vi "hdt_int_generator.vi"(9 "hdt.int.p.readParams":T2={"hdt.int.s.transferSource"=0, "hdt.int.p.useInternalMemStartPos"=FALSE, "hdt.int.p.memStartPos"=0.0, "hdt.int.p.readLength"=100, "hdt.int.p.readFwd"=TRUE, "hdt.int.p.memReadDec"=10, "hdt.int.p.startTransfer"=TRUE} {"hdt.int.s.transferSource" items=["memoryChan1", "memoryChan2", "processVarFixedNoPts", "processVarStream", "systemId", "interleaveMemCh1Ch2"]; "hdt.int.p.memReadDec" min=2}, 11 "hdt.int.p.memWriteSource":u8(ring) items=["ORT", "SICM"]) -> (0 "hdt.int.s.debug":T1)   [LabVIEW 2016]
uses:
  <vilib>/rvi/Emulation/niFpgaEmulationIsFPGAContextNoSignature.vi
  <vilib>/rvi/Emulation/niFpgaSctlEmulationGetInTimedLoop.vi
  <vilib>/rvi/errors/niFpgaSetErrorForExecOnDevCompSimple.vi
  <vilib>/rvi/eio/common/nirviEmuReportErrorAndStop.vi
  <vilib>/rvi/DataTransferAndStorage/Container/Common/niFpgaContainerGetUniqueNameForEmu.vi
  <vilib>/rvi/FIFO/Fifo_Resource/nirvififoEmulationSetSize.vi
  <vilib>/rvi/FIFO/Fifo_Resource/nirviFifoEmulationQueueMgr.vi
  <instcachedir>/0/nirviFifoEmulationQueueMgr_E5CAEC123FF24DC58D834DCA3CDAA9B5.lvgen/nirviFifoEmulationQueueMgr_E5CAEC123FF24DC58D834DCA3CDAA9B5_033.vi
  <vilib>/Utility/error.llb/Clear Errors.vi
  <vilib>/rvi/FIFO/Fifo_Resource/nirvififoEmulationCreateLock.vi
  <vilib>/rvi/Emulation/niFpgaProcessEmulError.vi
  <vilib>/rvi/FIFO/Fifo_Resource/nirvififoEmulationObtainLock.vi
  <vilib>/rvi/FIFO/Fifo_Resource/nirvififoEmulationReleaseLock.vi
  <vilib>/rvi/occurrence/nirviWaitOnOccurrenceBase.vi
  <vilib>/rvi/errors/nirviReportUnexpectedCaseInternalError.vi
  <vilib>/rvi/errors/nirviReportUnexpectedCaseInternalError (U32).vi
  <instcachedir>/0/nirviFifoEmulationQueueMgr_E5CAEC123FF24DC58D834DCA3CDAA9B5.lvgen/nirviFifoEmulationQueueMgr_E5CAEC123FF24DC58D834DCA3CDAA9B5_003.vi
  <vilib>/rvi/Memory/Memory_Emulation/nirvimemoryFastEmulation.vi
  <vilib>/rvi/Memory/Memory_Emulation/nirvimemoryEmulation.vi
  <instcachedir>/0/nirviFifoEmulationQueueMgr_E5CAEC123FF24DC58D834DCA3CDAA9B5.lvgen/nirviFifoEmulationQueueMgr_E5CAEC123FF24DC58D834DCA3CDAA9B5_009.vi
  <vilib>/rvi/FIFO/Fifo_Resource/nirvififoEmulationDetermineInputValidOut.vi
  <vilib>/rvi/DataTransferAndStorage/Container/XNode/niFpgaContainer.xnode
  <vilib>/rvi/FIFO/Fifo_Resource/nirvififoEmulationRead.vi
  <vilib>/rvi/DataTransferAndStorage/Handshake/Emulation/niFpgaHandshakeEmulation.vi
  <vilib>/rvi/FIFO/Fifo_Resource/nirvififoEmulationWrite.vi
  <instrlib>/_niInstr/Basic Elements/v1/FPGA/niInstr Basic Elements v1 FPGA.lvlib
panel:
  out "hdt.int.s.currentStagingEl":cluster{"Element":i16, "Output Valid":bool}
  out "hdt.int.s.storedMemPos":u16
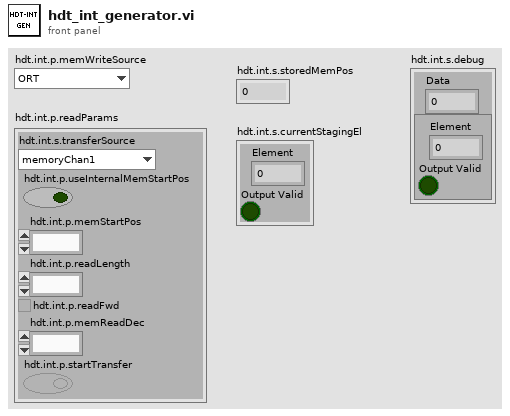
[diagram p1: front panel]
types:
  T1 = cluster{"Data":u16, cluster{"Element":i16, "Output Valid":bool}}
  T2 = cluster{"hdt.int.s.transferSource":u8, "hdt.int.p.useInternalMemStartPos":bool, "hdt.int.p.memStartPos":fxp<+,14,14>, "hdt.int.p.readLength":u16, "hdt.int.p.readFwd":bool, "hdt.int.p.memReadDec":u16, "hdt.int.p.startTransfer":bool}
  T3 = cluster{"Element":cluster{"address":u16, "interactionPair":cluster{"interaction":i16, "background":i16}}, "Output Valid":bool}
  T4 = cluster{"address":u16, "interactionPair":cluster{"interaction":i16, "background":i16}}
  T5 = cluster{"Element":cluster{"address":u16, "interactionPair":cluster{"interaction":i16, "background":i16}}, "Output Valid":bool}[]
  T6 = cluster{"interaction":i16, "Output Valid":bool}[]
  T7 = cluster{"Data":u16, cluster{"interaction":i16, "Output Valid":bool}}
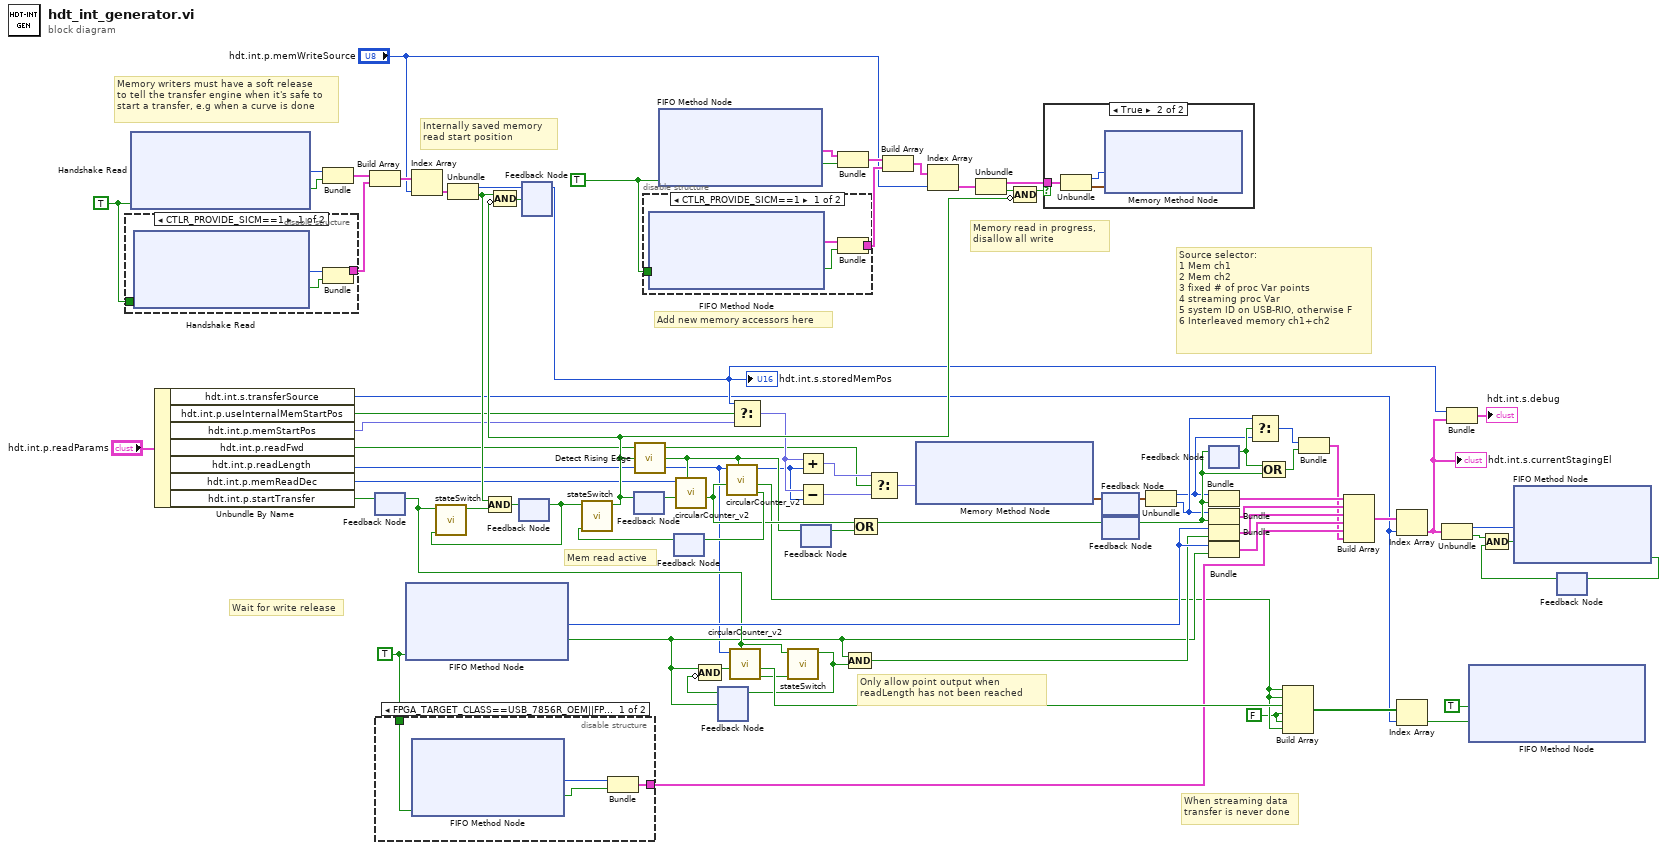
[diagram p0: block diagram]
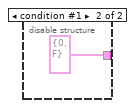
[diagram p2: hidden frame]
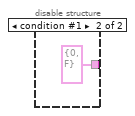
[diagram p3: hidden frame]
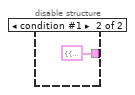
[diagram p4: hidden frame]
diagram:
  w3 = FALSE ("element")
  w45 = TRUE ("Ready for Output")
  w13 = TRUE ("Ready for Output")
  w46 = TRUE ("Ready for Output")
  # "Source selector:\n1 Mem ch1\n2 Mem ch2\n3 fixed # of proc Var points\n4 streaming proc Var\n5 system ID on USB-RIO, otherwise F\n6 Interleaved memory ch1+ch2"
  # "When streaming data\ntransfer is never done"
  # "Mem read active"
  # "Internally saved memory \nread start position"
  # "Memory writers must have a soft release\nto tell the transfer engine when it's safe to\nstart a transfer, e.g when a curve is done"
  # "Wait for write release"
  # "Only allow point output when readLength has not been reached"
  # "Memory read in progress,\ndisallow all write"
  # "Add new memory accessors here"
  n1 = disable-structure shown="CTLR_PROVIDE_SICM==1" {
    disable-tunnel: [w85 cluster{"Data":u16, "Output Valid":bool} {"Data"=0, "Output Valid"=FALSE}] -> w52
    disable-tunnel: w45 -> [w84 _]
    frame condition #0 (active) {
      n2 = xnode ("Handshake Read")("Ready for Output"=w84) -> ("Data"=w87:u16, "Output Valid"=w86:bool)  [unwired: 1 in, 1 out]
      n3 = Bundle("Data"=w87, "Output Valid"=w86) -> (w85:cluster{"Data":u16, "Output Valid":bool})  [unwired: 1 in]
    }
    frame condition #1 {
    }
  }
  n4 = xnode ("Handshake Read")("Ready for Output"=w45) -> ("Data"=w55:u16, "Output Valid"=w54:bool)  [unwired: 1 in, 1 out]
  n5 = Unbundle By Name("hdt.int.p.readParams") -> ("hdt.int.s.transferSource"=w30:u8, "hdt.int.p.useInternalMemStartPos"=w38:bool, "hdt.int.p.memStartPos"=w39:fxp<+,14,14>, "hdt.int.p.readFwd"=w15:bool, "hdt.int.p.readLength"=w14:u16, "hdt.int.p.memReadDec"=w37:u16, "hdt.int.p.startTransfer"=w36:bool)
  n6 = Bundle("Data"=w55, "Output Valid"=w54) -> (w53:cluster{"Data":u16, "Output Valid":bool})  [unwired: 1 in]
  n7 = Build Array(w53, w52) -> (w51:cluster{"Data":u16, "Output Valid":bool}[])
  n8 = feedback #1() -> (w24:bool)  [unwired: 1 in]
  n9 = feedback-in #1(w36) -> ()
  n10 = disable-structure shown="FPGA_TARGET_CLASS==USB_7856R_OEM||FPGA_TARGET_CLASS==USB_7856R" {
    disable-tunnel: w13 -> [w92 _]
    disable-tunnel: [w89 cluster{"Element":i16, "Output Valid":bool} {"Element"=0, "Output Valid"=FALSE} ("output cluster")] -> w12
    frame condition #0 (active) {
      n11 = xnode ("FIFO Method Node")("Ready for Output"=w92) -> ("Element"=w91:i16, "Output Valid"=w90:bool)  [unwired: 1 in, 1 out]
      n12 = Bundle("Element"=w91, "Output Valid"=w90) -> (w89:cluster{"Element":i16, "Output Valid":bool})  [unwired: 1 in]
    }
    frame condition #1 {
    }
  }
  n13 = xnode ("FIFO Method Node")("Ready for Output"=w13) -> ("Element"=w60:i16, "Output Valid"=w21:bool)  [unwired: 1 in, 1 out]
  n14 = Index Array(array=w51, index="hdt.int.p.memWriteSource") -> (element=w49:cluster{"Data":u16, "Output Valid":bool})
  n15 = Unbundle(w49) -> ("Data"=w48:u16, "Output Valid"=w43:bool)
  n16 = feedback #2() -> (w1:bool)  [unwired: 1 in]
  n17 = call "stateSwitch.vi"("disable"=w1, "enable"=w24) -> ("state"=w47:bool)  [unwired: 9 in]
  n18 = Compound Arithmetic op=AND(w43, w47) -> (w2:bool)
  n19 = feedback-in #2(w2) -> ()
  n20 = feedback #3() -> (w34:u16)  [unwired: 1 in]
  "hdt.int.s.storedMemPos" <- w34
  n21 = feedback #4() -> (w44:bool)  [unwired: 1 in]
  n22 = disable-structure shown="CTLR_PROVIDE_SICM==1" {
    disable-tunnel: [w95 T3 {"Element"={"address"=0, "interactionPair"={"interaction"=0, "background"=0}}, "Output Valid"=FALSE}] -> w75
    disable-tunnel: w46 -> [w94 _]
    frame condition #0 (active) {
      n23 = xnode ("FIFO Method Node")("Ready for Output"=w94) -> ("Element"=w97:T4, "Output Valid"=w96:bool)  [unwired: 1 in, 1 out]
      n24 = Bundle("Element"=w97, "Output Valid"=w96) -> (w95:T3)  [unwired: 1 in]
    }
    frame condition #1 {
    }
  }
  n25 = xnode ("FIFO Method Node")("Ready for Output"=w46) -> ("Element"=w82:T4, "Output Valid"=w81:bool)  [unwired: 1 in, 1 out]
  n26 = feedback #5() -> (w66:bool)  [unwired: 1 in]
  n27 = call "stateSwitch.vi"("disable"=w66, "enable"=w1) -> ("state"=w42:bool)  [unwired: 9 in]
  n28 = Compound Arithmetic op=AND(w43, invert w42) -> (w41:bool)
  n29 = feedback-in #3(w48, w41) -> ()
  n30 = feedback-in #4(w42) -> ()
  n31 = call <instrlib>:"Detect Rising Edge.vi"("signal"=w42) -> ("edge detected"=w26:bool)  [unwired: 14 in]
  n32 = call "circularCounter_v2.vi"("reset"=w26, "doStep"=w44, "maxCount"=w37) -> ("maxPulse"=w32:bool)  [unwired: 5 in, 3 out]
  n33 = feedback #6() -> (w57:bool)  [unwired: 1 in]
  n34 = Compound Arithmetic op=AND(w21, invert w57) -> (w58:bool)
  n35 = call "circularCounter_v2.vi"("reset"=w26, "doStep"=w32, "maxCount"=w14) -> ("maxReached"=w67:bool, "maxPulse"=w4:bool, "index"=w18:u16)  [unwired: 5 in, 1 out]
  n36 = feedback-in #5(w67) -> ()
  n37 = call "circularCounter_v2.vi"("reset"=w24, "doStep"=w58, "maxCount"=w14) -> ("maxReached"=w22:bool, "maxPulse"=w23:bool)  [unwired: 5 in, 2 out]
  n38 = Select(t=w34, s=w38, f=w39) -> (s? t:f=w19:fxp<+,16,16>)
  n39 = call "stateSwitch.vi"("disable"=w22, "enable"=w24) -> ("state"=w20:bool)  [unwired: 9 in]
  n40 = feedback-in #6(w20, w21) -> ()
  n41 = Add(x=w19, y=w18) -> (x+y=w68:fxp<+,14,14>)
  n42 = Subtract(x=w19, y=w18) -> (x-y=w16:fxp<+,14,14>)
  n43 = feedback-in #7(w26) -> ()
  n44 = feedback #7() -> (w25:bool)  [unwired: 1 in]
  n45 = Bundle("Element"=w82, "Output Valid"=w81) -> (w80:T3)  [unwired: 1 in]
  n46 = Compound Arithmetic op=AND(w21, w20) -> (w56:bool)
  n47 = Compound Arithmetic op=OR(w32, w25) -> (w27:bool)
  n48 = Select(t=w68, s=w15, f=w16) -> (s? t:f=w17:fxp<+,14,14>)
  n49 = Build Array(w80, w75) -> (w83:T5)
  n50 = xnode ("Memory Method Node")("Address"=w17) -> ("Data"=w73:cluster{"interaction":i16, "background":i16})  [unwired: 1 in, 1 out]
  n51 = Index Array(array=w83, index="hdt.int.p.memWriteSource") -> (element=w79:T3)
  n52 = Unbundle(w79) -> ("Element"=w77:T4, "Output Valid"=w78:bool)
  n53 = Compound Arithmetic op=AND(w78, invert w42) -> (w76:bool)
  n54 = case shown="True" w76 {
    tunnel: w77 -> [_ w101]
    frame False {
    }
    frame True {
      n55 = Unbundle(w101) -> ("address"=w100:u16, "interactionPair"=w99:cluster{"interaction":i16, "background":i16})
      n56 = xnode ("Memory Method Node")("Address"=w100, "Data"=w99) -> ()  [unwired: 1 in, 1 out]
    }
  }
  n57 = feedback #8() -> (w65:cluster{"interaction":i16, "background":i16})  [unwired: 1 in]
  n58 = feedback-in #8(w73) -> ()
  n59 = feedback #9() -> (w9:bool)  [unwired: 1 in]
  n60 = feedback-in #9(w27) -> ()
  n61 = Unbundle(w65) -> ("interaction"=w5:i16, "background"=w6:i16)
  n62 = feedback-in #10(w9) -> ()
  n63 = feedback #10() -> (w10:bool)  [unwired: 1 in]
  n64 = Bundle("interaction"=w5, w9) -> (w72:cluster{"interaction":i16, bool})  [unwired: 1 in]
  n65 = Bundle("background"=w6, w9) -> (w71:cluster{"background":i16, bool})  [unwired: 1 in]
  n66 = Bundle("Element"=w60, w56) -> (w61:cluster{"Element":i16, bool})  [unwired: 1 in]
  n67 = Bundle("Element"=w60, "Output Valid"=w21) -> (w59:cluster{"Element":i16, "Output Valid":bool})  [unwired: 1 in]
  n68 = Select(t=w6, s=w10, f=w5) -> (s? t:f=w11:i16)
  n69 = Compound Arithmetic op=OR(w10, w9) -> (w8:bool)
  n70 = Build Array(w4, w4, w23, w3, w3, w4) -> (w31:bool[])
  n71 = Bundle("interaction"=w11, w8) -> (w7:cluster{"interaction":i16, bool})  [unwired: 1 in]
  n72 = Build Array(w72, w71, w61, w59, w12, w7) -> (w74:T6)
  n73 = Index Array(array=w74, index=w30) -> (element=w35:cluster{"interaction":i16, "Output Valid":bool})
  "hdt.int.s.currentStagingEl" <- w35
  n74 = Index Array(array=w31, index=w30) -> (element=w29:bool)
  n75 = Unbundle(w35) -> ("interaction"=w70:i16, "Output Valid"=w69:bool)
  n76 = Bundle("Data"=w34, w35) -> (→"hdt.int.s.debug":T7)  [unwired: 1 in]
  n77 = xnode ("FIFO Method Node")("Element"=TRUE, "Input Valid"=w29) -> ()  [unwired: 1 in, 2 out]
  n78 = feedback #11() -> (w62:bool)  [unwired: 1 in]
  n79 = Compound Arithmetic op=AND(w69, w62) -> (w64:bool)
  n80 = xnode ("FIFO Method Node")("Element"=w70, "Input Valid"=w64) -> ("Ready for Input"=w63:bool)  [unwired: 1 in, 1 out]
  n81 = feedback-in #11(w63) -> ()
